vi "ShowRobotPosition.vi"() -> ()   [LabVIEW 2009, in "Host.lvlib"]
uses:
  Host.lvlib
  <vilib>/vision/Image Controls.llb/IMAQ Image.ctl
  NetworkVarTarget.lvlib
  Draw.lvlib
panel:
  out "RobotPosition_fromDrive":cluster{"X":dbl, "Y":dbl, "Angle":dbl}
  out "Image Out":T1(plugin-control)
  in  "Set goal":bool
  out "Robot Position":cluster{"X":dbl, "Y":dbl, "Angle":dbl}
  in  "Goal":cluster{"X":dbl, "Y":dbl}
  out "Map":picture
  in  "stop":bool
  in  "Reset Map":bool
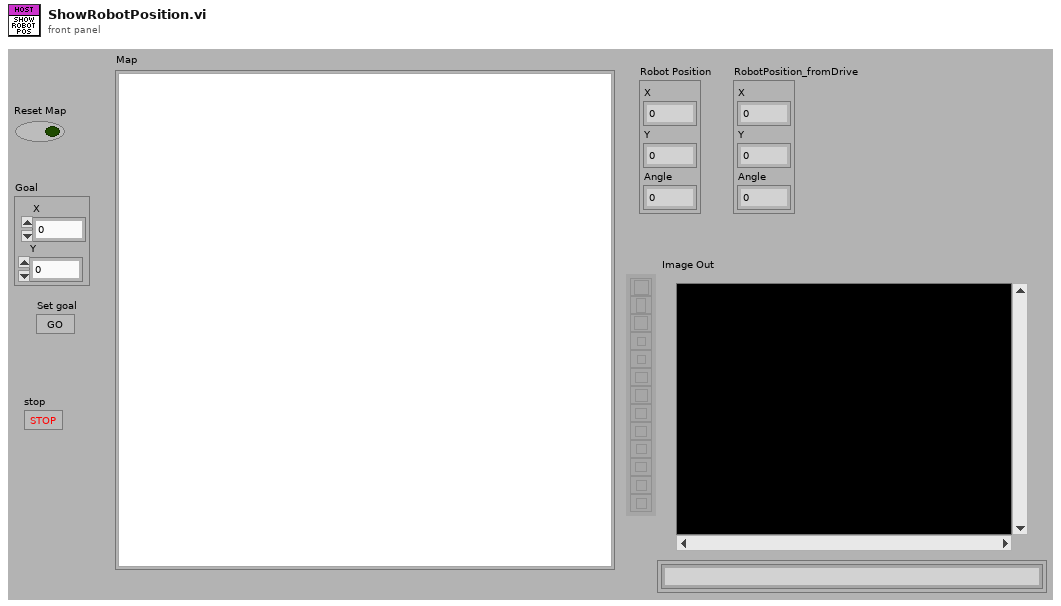
[diagram p1: front panel]
types:
  T1 = typedef "IMAQ Image.ctl" = refnum<image>
  T2 = cluster{"Position":cluster{"X":dbl, "Y":dbl, "Angle":dbl}, "Speed":cluster{"Left":dbl, "Right":dbl}}
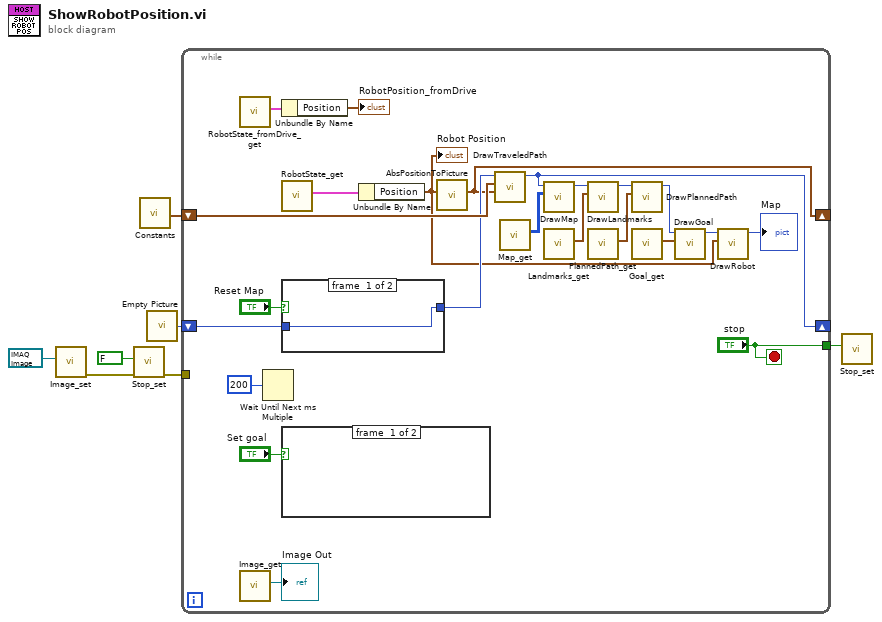
[diagram p0: block diagram]
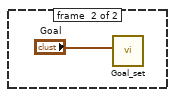
[diagram p2: hidden frame]
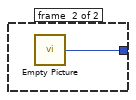
[diagram p3: hidden frame]
diagram:
  n1 = call "Image_set.vi"("Image"=T1 refnum) -> ("error out"=w2:errorcluster)  [unwired: 10 in]
  n2 = call "Stop_set.vi"("error in (no error)"=w2, "Stop? (F)"=FALSE ("Stop")) -> ("error out"=w6:errorcluster)  [unwired: 9 in]
  n3 = call "Constants.vi"() -> ("PictureCenterPoint"=w3:cluster{"x":i16, "y":i16})  [unwired: 16 in, 3 out]
  n4 = call "Empty Picture"() -> ("empty picture"=w7:picture)
  n5 = while {
    shift-right: [w14] -> _
    shift-left: w7 -> [w28]
    shift-right: [w20] -> _
    shift-left: w3 -> [w22]
    tunnel: w6 -> [_]
    tunnel: ["stop"] -> w4
    stop <- "stop" stop-if-true
    n6 = call "RobotState_fromDrive_get.vi"() -> ("RobotState_fromDrive"=w9:T2)  [unwired: 10 in, 1 out]
    n7 = call "Image_get.vi"() -> ("Image Out"=→"Image Out":T1)  [unwired: 10 in, 1 out]
    n8 = Wait Until Next ms Multiple(millisecond multiple=u32 200) -> ()  [unwired: 1 out]
    n9 = Unbundle By Name(w9) -> ("Position"=→"RobotPosition_fromDrive":cluster{"X":dbl, "Y":dbl, "Angle":dbl})
    n10 = call "RobotState_get.vi"() -> ("RobotState"=w26:T2)  [unwired: 10 in, 1 out]
    n11 = case shown="False" "Reset Map" {
      tunnel: w28 -> [w32 _]
      tunnel: [w32 w33] -> w21
      frame #0 {
      }
      frame #1 {
        n12 = call "Empty Picture"() -> ("empty picture"=w33:picture)
      }
    }
    n13 = case shown="True" "Set goal" {
      frame #0 {
      }
      frame #1 {
        n14 = call "Goal_set.vi"("Goal"="Goal") -> ()  [unwired: 10 in, 1 out]
      }
    }
    n15 = Unbundle By Name(w26) -> ("Position"=w19:cluster{"X":dbl, "Y":dbl, "Angle":dbl})
    "Robot Position" <- w19
    n16 = call "AbsPositionToPicture.vi"("input position"=w19) -> ("output point"=w20:cluster{"x":i16, "y":i16})  [unwired: 10 in]
    n17 = call "DrawTraveledPath.vi"("end point"=w20, "start point"=w22, "picture"=w21) -> ("new picture"=w14:picture)  [unwired: 7 in, 1 out]
    n18 = call "Map_get.vi"() -> ("Map"=w13:i8[][])  [unwired: 10 in, 1 out]
    n19 = call "DrawMap.vi"("Map"=w13, "picture"=w14) -> ("new picture"=w12:picture)  [unwired: 8 in, 1 out]
    n20 = call "Landmarks_get.vi"() -> ("Landmarks"=w10:cluster{"X position":dbl, "Y position":dbl}[])  [unwired: 10 in, 1 out]
    n21 = call "DrawLandmarks.vi"("Landmarks"=w10, "picture"=w12) -> ("new picture"=w11:picture)  [unwired: 8 in, 1 out]
    n22 = call "PlannedPath_get.vi"() -> ("PlannedPath"=w15:cluster{"X position":dbl, "Y position":dbl}[])  [unwired: 10 in, 1 out]
    n23 = call "DrawPlannedPath.vi"("path points"=w15, "picture"=w11) -> ("new picture"=w18:picture)  [unwired: 8 in, 1 out]
    n24 = call "Goal_get.vi"() -> ("Goal"=w16:cluster{"X":dbl, "Y":dbl})  [unwired: 10 in, 1 out]
    n25 = call "DrawGoal.vi"("point"=w16, "picture"=w18) -> ("new picture"=w17:picture)  [unwired: 8 in, 1 out]
    n26 = call "DrawRobot.vi"("RobotPosition (m and rad)"=w19, "picture"=w17) -> ("new picture"=→"Map":picture)  [unwired: 8 in, 1 out]
  }
  n27 = call "Stop_set.vi"("Stop? (F)"=w4) -> ()  [unwired: 10 in, 1 out]
